vi "cálculo Br Cr.vi"(8 "Resolución":i32, 9 "Número de índices de refracción":i32=4, 10 "npr":cdb[](array[numeric])=[1.7494752407073975+0.0i, 86.81378173828125+0.0i, 0.1659284383058548-3.1242640018463135i, 0.1731347292661667-2.9031877517700195i, 3.5999114513397217-4.32273006439209i, 3.6872870922088623-4.200350761413574i, 1.5319026708602905+0.0i, 5.381030245572629e-17+0.8788179159164429i], 11 "Matrices interfaces":T1=[[1.0+0.0i, 0.0+0.0i], [0.0+0.0i, 1.0+0.0i], [1.0+0.0i, 0.0+0.0i], [0.0+0.0i, 1.0+0.0i], [2.6596293880104103+0.1933537734864808i, -0.024770245793668728+0.7905295424518692i], [1.0607287655039235-7.668932008898614i, 2.6596293880104103+0.1933537734864808i], [2.989409851222815+0.2053102271642363i, -0.01706752823955897+0.971719429141639i], [1.1201972468486874-8.143850714546906i, 2.989409851222815+0.2053102271642363i], [1.0003383845711877+0.001534851791733266i, 0.0001707502361469053+0.009965964768471348i], [0.3091918105040684-0.06238566122364114i, 1.0003383845711877+0.001534851791733266i], [1.0004232271100613+0.0015348951915381635i, 0.000698047230901286+0.010073200586728453i], [0.3092005298064502-0.06238740696414413i, 1.0004232271100613+0.0015348951915381635i], [1.0+0.0i, 0.0+0.0i], [0.0+0.0i, 1.0+0.0i], [1.0+0.0i, 0.0+0.0i], [0.0+0.0i, 1.0+0.0i]]) -> (1 "1\nnpr3":cdb[][][](array[numeric]), 2 "Br\nCr":cdb[][][](array[numeric]), 3 "npr3":cdb[](array[numeric]), 5 "Vetor matrices":cdb[][][][](array[numeric]))   [LabVIEW 2025]
uses:
  <vilib>/Analysis/Matrix/Datatypes/ComplexMatrix.ctl
  <vilib>/Analysis/baseanly.llb/Complex A x B.vi
  <vilib>/Analysis/Matrix/Numeric/Conversions/Array To Matrix - CA2.vi
  <vilib>/Analysis/NI_AALBase.lvlib
  <vilib>/Analysis/Matrix/NI_Matrix.lvlib
panel:
  out "Vector C":cdb[][][][](array[numeric]) caption="Array"
  # "Salidas"
  # "Entradas"
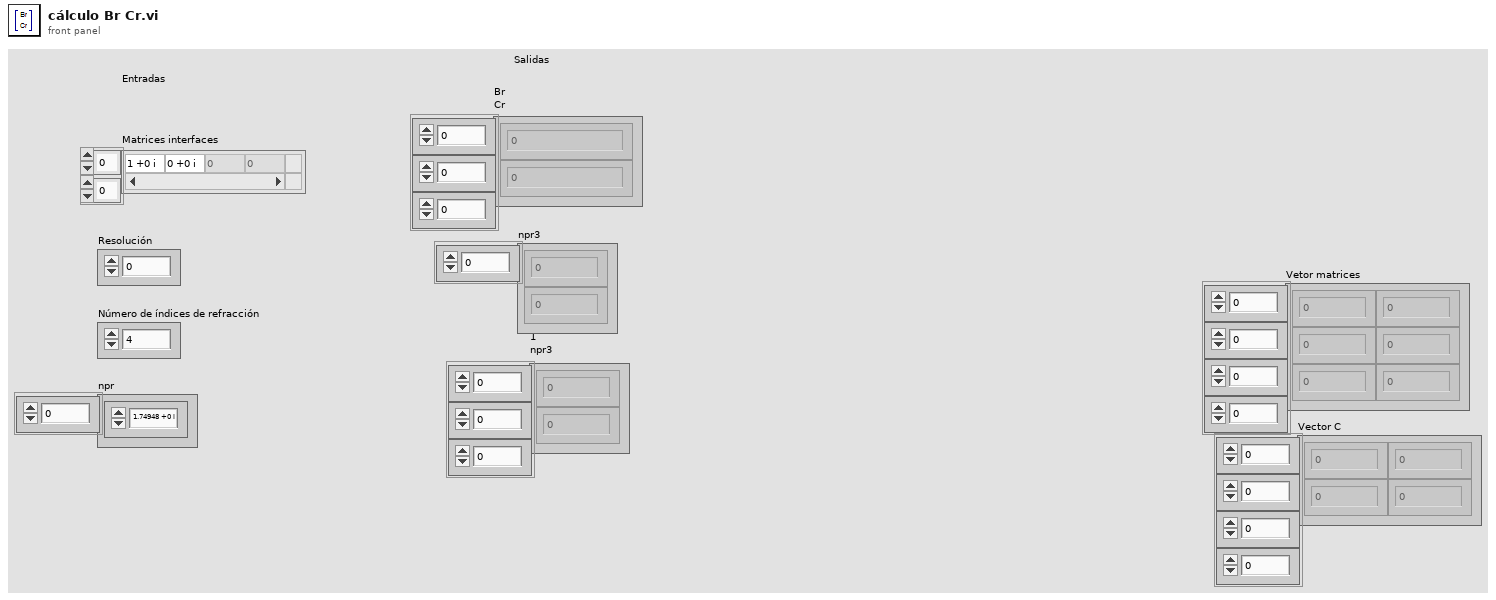
[diagram p1: front panel]
types:
  T1 = typedef "NI_Matrix.lvlib/ComplexMatrix.ctl" = cdb[][]
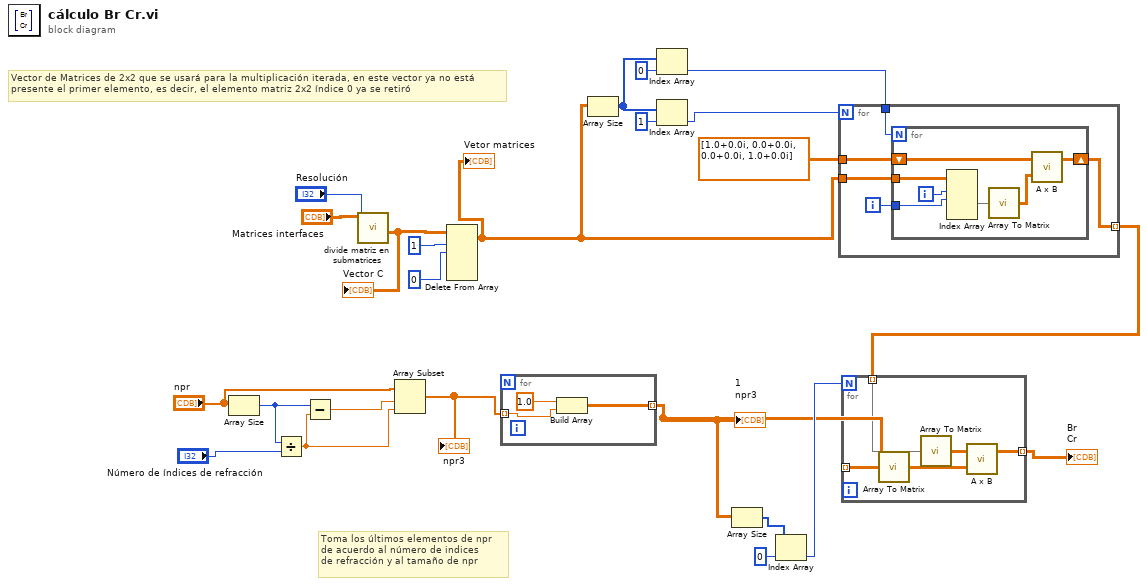
[diagram p0: block diagram]
diagram:
  # "Toma los últimos elementos de npr\nde acuerdo al número de indices\nde refracción y al tamaño de npr"
  # "Vector de Matrices de 2x2 que se usará para la multiplicación iterada, en este vector ya no está\npresente el primer elemento, es decir, el elemento matriz 2x2 índice 0 ya se retiró"
  n1 = Array Size(array="npr") -> (size(s)=w20:i32)
  n2 = Divide(x=w20, y="Número de índices de refracción") -> (x/y=w19:dbl)
  n3 = Subtract(x=w20, y=w19) -> (x-y=w18:dbl)
  n4 = call "divide matriz en submatrices.vi"("Resolución"="Resolución", "Matriz compleja  A"="Matrices interfaces") -> ("Vector C"=w17:cdb[][][][])  [unwired: 6 in, 3 out]
  "Vector C" <- w17
  n5 = Array Subset(array="npr", index=w18, length=w19) -> (w16:cdb[])
  "npr3" <- w16
  n6 = Delete From Array(array=w17, length=1, index (dim 0)=0 ("index (page)")) -> (array with subset deleted=w6:cdb[][][][])  [unwired: 3 in, 1 out]
  "Vetor matrices" <- w6
  n7 = for {
    tunnel: w16 -> [w26] mode=indexing
    tunnel: [w25] -> w2 mode=indexing
    n8 = Build Array(1.0, w26) -> (w25:T1)
  }
  "1\nnpr3" <- w2
  n9 = Array Size(array=w6) -> (size(s)=w11:i32[])
  n10 = Index Array(array=w11, index=0) -> (element=w8:i32)
  n11 = Index Array(array=w11, index=1) -> (element=w7:i32)
  n12 = Array Size(array=w2) -> (size(s)=w14:i32[])
  n13 = Index Array(array=w14, index=0) -> (element=w12:i32)
  n14 = for {
    N: w7 -> [_]
    tunnel: w8 -> [w32]
    tunnel: w6 -> [w31]
    tunnel: T1 [[1.0+0.0i, 0.0+0.0i], [0.0+0.0i, 1.0+0.0i]] ("Complex Matrix 2") -> [w29]
    tunnel: [w28] -> w3 mode=indexing
    i -> [w30]
    n15 = for {
      N: w32 -> [_]
      tunnel: w31 -> [w39]
      tunnel: w30 -> [w37]
      shift-right: [w33] -> w28
      shift-left: w29 -> [w34]
      i -> [w38]
      n16 = Index Array(array=w39, index (dim 0)=w38, index (dim 1)=w37) -> (element=w36:cdb[][])  [unwired: 2 in]
      n17 = call-poly <vilib>:"Array To Matrix.vi"("Complex 2D Array"=w36) -> ("Complex Matrix"=w35:T1)
      n18 = call-poly <vilib>:"A x B.vi"("B"=w35, "A"=w34) -> ("A x B"=w33:T1)  [unwired: 1 out]
    }
  }
  n19 = for {
    N: w12 -> [_]
    tunnel: w3 -> [w44] mode=indexing
    tunnel: w2 -> [w43] mode=indexing
    tunnel: [w40] -> w1 mode=indexing
    n20 = call-poly <vilib>:"Array To Matrix.vi"("Complex 2D Array"=w43) -> ("Complex Matrix"=w41:T1)
    n21 = call-poly <vilib>:"Array To Matrix.vi"("Complex 2D Array"=w44) -> ("Complex Matrix"=w42:T1)
    n22 = call-poly <vilib>:"A x B.vi"("B"=w41, "A"=w42) -> ("A x B"=w40:T1)  [unwired: 1 out]
  }
  "Br\nCr" <- w1
